vi "Get X Y and Cost.vi"(11 "OccupancyGridMapNode in":refnum<class "NI_Robotics_OccupancyGridMapNode.lvclass">) -> (0 "Cost":dbl, 1 "y":i32, 2 "x":i32, 3 "OccupancyGridMapNode out":refnum<class "NI_Robotics_OccupancyGridMapNode.lvclass">)   [LabVIEW 2017, in "NI_Robotics_OccupancyGridMapNode.lvclass"]
uses:
  <vilib>/robotics/Navigation/shared/MapNode/OccupancyGridNode/NI_Robotics_OccupancyGridMapNode.lvclass
  <vilib>/robotics/Navigation/shared/MapNode/OccupancyGridNode/NI_Robotics_OccupancyGridMapNode.lvclass/NI_Robotics_OccupancyGridMapNode.ctl
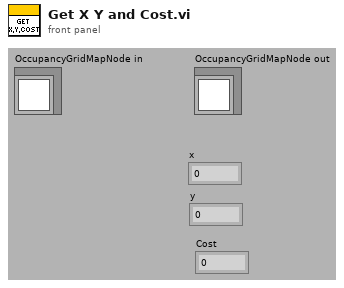
[diagram p1: front panel]
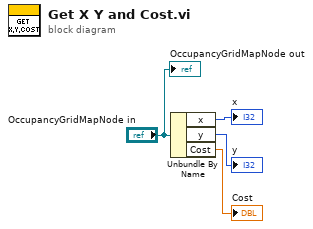
[diagram p0: block diagram]
diagram:
  n1 = Unbundle By Name("OccupancyGridMapNode in") -> ("x"=→"x":i32, "y"=→"y":i32, "Cost"=→"Cost":dbl)
  "OccupancyGridMapNode out" <- "OccupancyGridMapNode in"
